vi "CurrentSetX.vi"(10 "Cluster":T1={"VISA resource name"="COM6", "baud rate (9600)"=9600, "data bits (8)"=8, "parity (0:none)"=enum."None"} {"data bits (8)" min=5 max=8 step=1}, 11 "电流设置":dbl min=-5.0 max=5.0 step=0.2) -> ()   [LabVIEW 2020, in "YP03-60CurrentSource_1.lvlib"]
uses:
  Libraries/YP03-60CurrentSource_1/YP03-60CurrentSource_1.lvlib
  <vilib>/Instr/_visa.llb/VISA Configure Serial Port (Instr).vi
panel:
  out "error out":errorcluster
  in  "error in (no error)":errorcluster
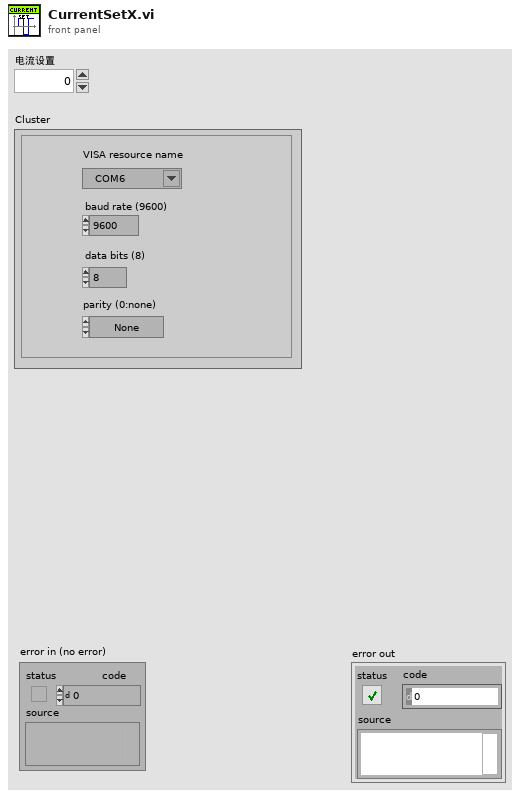
[diagram p1: front panel]
types:
  T1 = cluster{"VISA resource name":refnum<visa-resource-name>, "baud rate (9600)":u32, "data bits (8)":u16, "parity (0:none)":enum16{"None", "Odd", "Even", "Mark", "Space"}}
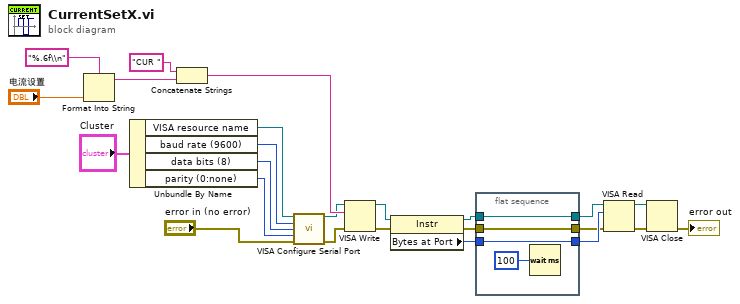
[diagram p0: block diagram]
diagram:
  n1 = Format Into String(format string="%.6f\\n", "电流设置") -> (resulting string=w21:string)  [unwired: 2 in, 1 out]
  n2 = Unbundle By Name("Cluster") -> ("VISA resource name"=w4:refnum<visa-resource-name>, "baud rate (9600)"=w3:u32, "data bits (8)"=w2:u16, "parity (0:none)"=w1:enum16{"None", "Odd", "Even", "Mark", "Space"})
  n3 = Concatenate Strings("CUR " ("string"), w21) -> (w17:string)
  n4 = call-poly "VISA Configure Serial Port"("VISA resource name"=w4, "baud rate (9600)"=w3, "data bits (8)"=w2, "parity (0:none)"=w1, "error in (no error)"="error in (no error)") -> ("VISA resource name out"=w10:refnum<visa-resource-name>, "error out"=w9:errorcluster)  [unwired: 9 in]
  n5 = VISA Write(VISA resource name=w10, write buffer=w17, error in (no error)=w9) -> (VISA resource name out=w19:refnum<visa-resource-name>, error out=w18:errorcluster)  [unwired: 1 out]
  n6 = property class="Instr"(reference=w19, error in=w18) -> (reference out=w14:refnum<visa-resource-name>, error out=w12:errorcluster, "Bytes at Port"=w16:u32)
  n7 = flat-sequence {
    tunnel: w14 -> [w28]
    tunnel: [w28] -> w13
    tunnel: [w27] -> w11
    tunnel: w12 -> [w27]
    tunnel: [w26] -> w15
    tunnel: w16 -> [w26]
    frame #0 {
      n8 = Wait (ms)(milliseconds to wait=u32 100) -> ()  [unwired: 1 out]
    }
  }
  n9 = VISA Read(VISA resource name=w13, byte count=w15, error in (no error)=w11) -> (VISA resource name out=w6:refnum<visa-resource-name>, error out=w7:errorcluster)  [unwired: 2 out]
  n10 = VISA Close(VISA resource name=w6, error in (no error)=w7) -> (error out=→"error out":errorcluster)
